vi "Get Pixel Format.vi"(8 "error in":errorcluster, 11 "Generic Image in":refnum<class "Generic Image.lvclass">) -> (0 "error out":errorcluster, 2 "Pixel Format":T1, 3 "Generic Image out":refnum<class "Generic Image.lvclass">)   [LabVIEW 2025, in "Generic Image.lvclass"]
uses:
  Generic Image.lvclass
  Pixel Format.ctl
  Generic Image.lvclass/Generic Image.ctl
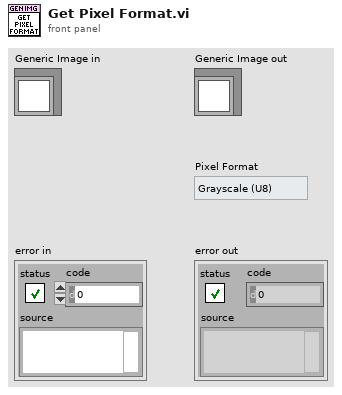
[diagram p1: front panel]
types:
  T1 = typedef "Generic Image.lvclass/Pixel Format.ctl" = enum16{"Grayscale (U8)", "Grayscale (I16)", "Grayscale (SGL)", "Complex (CSG)", "RGB (U32)", "HSL (U32)", "RGB (U64)", "Grayscale (U16)"}
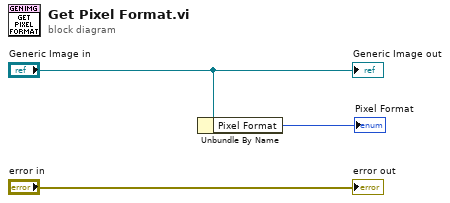
[diagram p0: block diagram]
diagram:
  n1 = Unbundle By Name("Generic Image in") -> ("Pixel Format"=→"Pixel Format":T1)
  "error out" <- "error in"
  "Generic Image out" <- "Generic Image in"
